vi "Destroy.vi"(8 "Error In":errorcluster, 11 "reference in":refnum<class "Reply Protocol Manager.lvclass">) -> (0 "Error Out":errorcluster, 3 "reference out":refnum<class "Reply Protocol Manager.lvclass">)   [LabVIEW 2023, in "HAL GOOP4.lvlib" / "Reply Protocol Manager.lvclass"]
uses:
  Reply Protocol Manager.lvclass
  Reply Protocol Manager.lvclass/Reply Protocol Manager.ctl
  Reply Protocol/Reply Protocol Base/Reply Protocol Base.lvclass
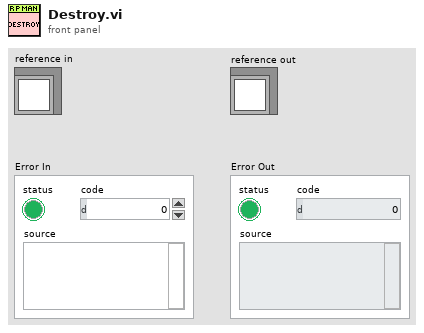
[diagram p1: front panel]
types:
  T1 = typedef "HAL GOOP4.lvlib/Reply Protocol Manager.lvclass/ObjectAttributes.ctl" = cluster{"Reply Protocols":map{string, refnum<class "Reply Protocol Base.lvclass">}}
  T2 = map{string, refnum<class "Reply Protocol Base.lvclass">}
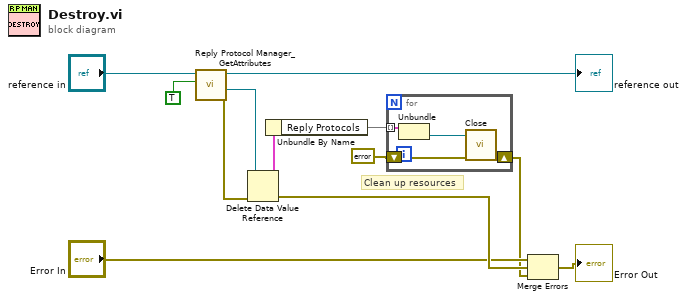
[diagram p0: block diagram]
diagram:
  # "Clean up resources"
  n1 = call "Reply Protocol Manager_GetAttributes.vi"("OnlyGetDvrReference(False)"=TRUE, "reference in"="reference in") -> ("Error Out"=w9:errorcluster, "DataRef"=w8:refnum<data-value>, "reference out"=→"reference out":refnum<class "Reply Protocol Manager.lvclass">)  [unwired: 6 in, 1 out]
  n2 = Delete Data Value Reference(data value reference=w8, error in=w9) -> (data value=w4:T1, error out=w7:errorcluster)
  n3 = Unbundle By Name(w4) -> ("Reply Protocols"=w3:T2)
  n4 = for {
    tunnel: w3 -> [w16] mode=indexing
    shift-right: [w14] -> w1
    shift-left: errorcluster {"status"=FALSE, "code"=0, "source"=""} ("error out") -> [w13]
    n5 = Unbundle(w16) -> ("Reply Protocol Base"=w15:refnum<class "Reply Protocol Base.lvclass">)  [unwired: 1 out]
    n6 = call-dynamic "Close.vi"("error in (no error)"=w13, "Reply Protocol Base in"=w15) -> ("error out"=w14:errorcluster)  [unwired: 8 in, 1 out]
  }
  n7 = Merge Errors("Error In", w7, w1) -> (→"Error Out":errorcluster)
